vi "IsmaTest_V2.vi"() -> ()   [LabVIEW 2017]
uses:
  BERTTA.dll
panel:
  out "pumpCTRL":dbl
  out "elapsed":dbl
  out "time_to_target":dbl
  out "Boolean 9":bool
  out "Boolean 8":bool
  out "Boolean 7":bool
  out "Boolean 6":bool
  out "Boolean 5":bool
  out "Boolean 4":bool
  out "Boolean 3":bool
  out "Boolean 2":bool
  out "Boolean":bool
  in  "Setpoint_W   /   Setpoint_T":dbl[][](array[numeric])
  in  "Pause":bool
  in  "Reset":bool
  in  "Manual":bool
  in  "Enable":bool
  in  "FR_manual":dbl
  out "FR":dbl(graph)
  out "paramsIn":dbl[](array[numeric])
  out "paramsOut":dbl[](array[numeric])
  out "RPM":dbl
  out "Weight":dbl
  in  "port_isma":i32=7
  in  "port":i32=4
  # "STOP"
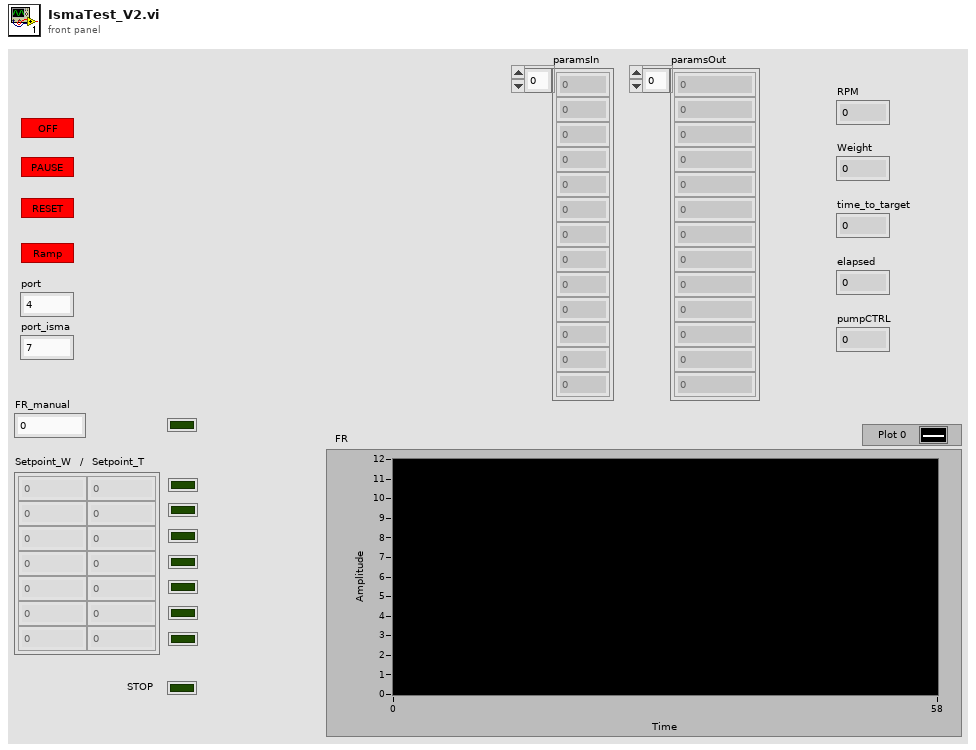
[diagram p1: front panel]
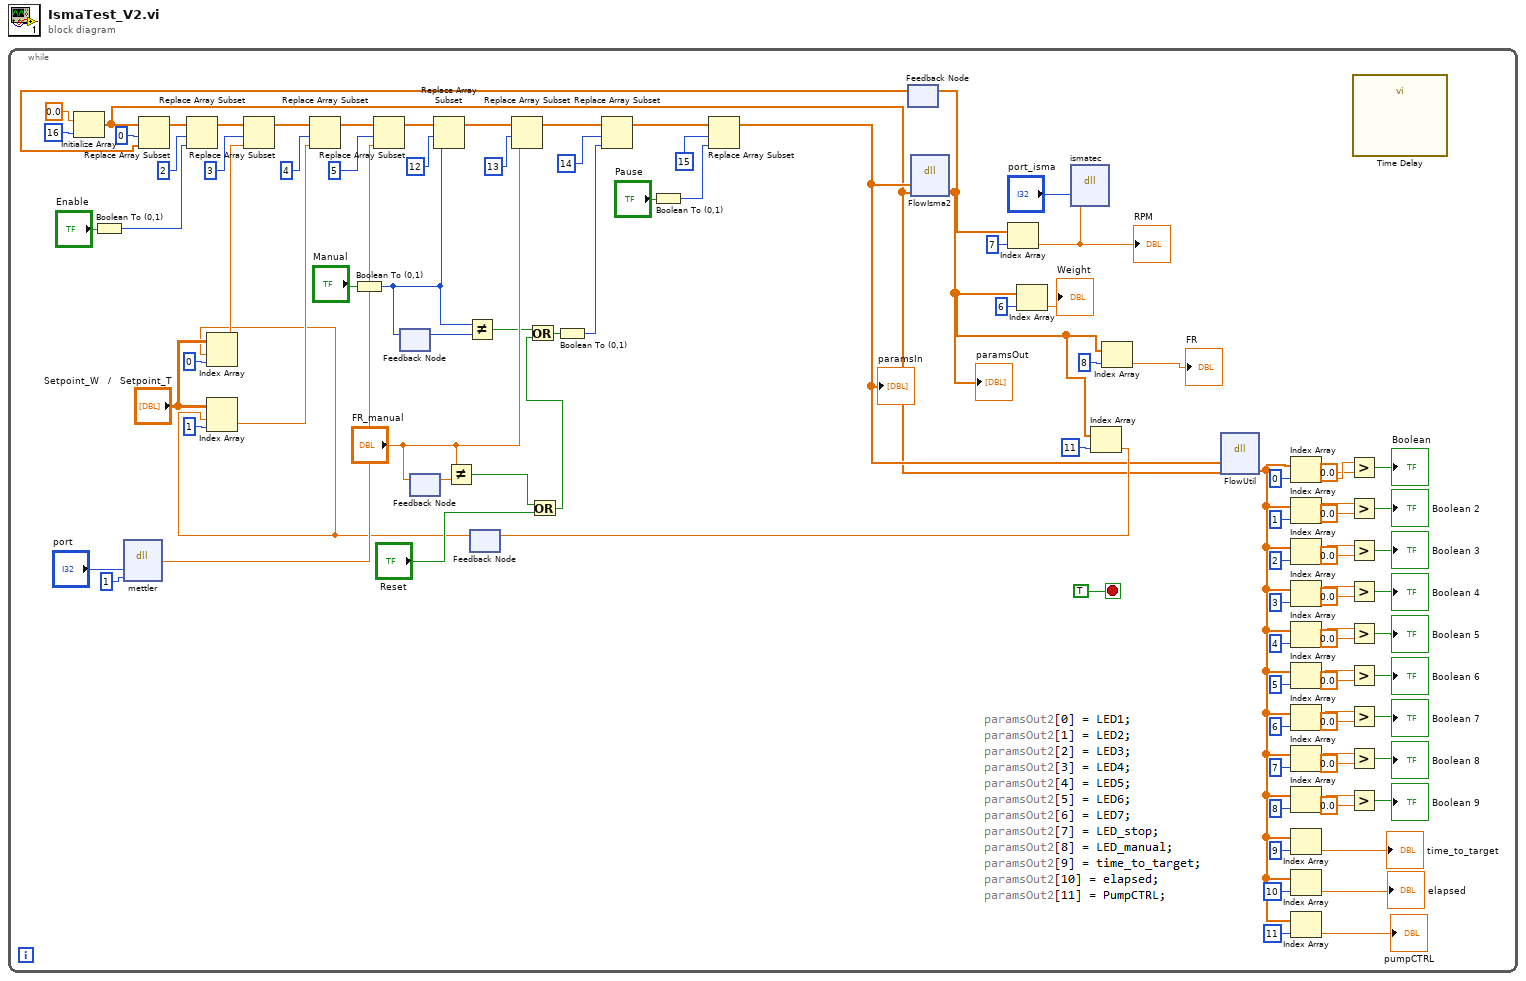
[diagram p0: block diagram]
diagram:
  n1 = while {
    stop <- TRUE stop-if-true
    n2 = Initialize Array(0.0 ("element"), 16 ("dimension size")) -> (w1:dbl[])
    n3 = Boolean To (0,1)(Boolean="Enable") -> (0, 1=w73:i16)
    n4 = dll-call lib="C:/Users/shresplab/OneDrive - Kemira Oyj/Documents/GitHub/Bertta/BERTTA/x64/Debug/BERTTA.dll" fn="mettler"("port"="port", "msg"=1) -> ("return type"=w90:dbl)  [unwired: 5 in, 2 out]
    n5 = Boolean To (0,1)(Boolean="Manual") -> (0, 1=w64:i16)
    n6 = feedback #1() -> (w65:i16)  [unwired: 1 in]
    n7 = feedback-in #1(w64) -> ()
    n8 = feedback #2() -> (w68:dbl)  [unwired: 1 in]
    n9 = feedback-in #2("FR_manual") -> ()
    n10 = Not Equal?(x="FR_manual", y=w68) -> (x != y?=w67:bool)
    n11 = Not Equal?(x=w64, y=w65) -> (x != y?=w61:bool)
    n12 = feedback #3() -> (w46:dbl)  [unwired: 1 in]
    n13 = Index Array(array="Setpoint_W   /   Setpoint_T", index (row)=w46, index (col)=0 ("disabled index (col)")) -> (element=w53:dbl)
    n14 = Index Array(array="Setpoint_W   /   Setpoint_T", index (row)=w46, index (col)=1 ("disabled index (col)")) -> (element=w50:dbl)
    n15 = Or(x=w67, y="Reset") -> (x .or. y?=w60:bool)
    n16 = Or(x=w61, y=w60) -> (x .or. y?=w63:bool)
    n17 = Boolean To (0,1)(Boolean=w63) -> (0, 1=w62:i16)
    n18 = Boolean To (0,1)(Boolean="Pause") -> (0, 1=w55:i16)
    n19 = feedback #4() -> (w82:dbl[])  [unwired: 1 in]
    n20 = Replace Array Subset(array=w1, new element=w82, index=0) -> (w81:dbl[])
    n21 = Replace Array Subset(array=w81, new element=w73, index=2) -> (w95:dbl[])
    n22 = Replace Array Subset(array=w95, new element=w53, index=3) -> (w93:dbl[])
    n23 = Replace Array Subset(array=w93, new element=w50, index=4) -> (w91:dbl[])
    n24 = Replace Array Subset(array=w91, new element=w90, index=5) -> (w78:dbl[])
    n25 = Replace Array Subset(array=w78, new element=w64, index=12) -> (w75:dbl[])
    n26 = Replace Array Subset(array=w75, new element="FR_manual", index=13) -> (w70:dbl[])
    n27 = Replace Array Subset(array=w70, new element=w62, index=14) -> (w57:dbl[])
    n28 = Replace Array Subset(array=w57, new element=w55, index=15) -> (w45:dbl[])
    "paramsIn" <- w45
    n29 = dll-call lib="C:/Users/shresplab/OneDrive - Kemira Oyj/Documents/GitHub/Bertta/BERTTA/x64/Debug/BERTTA.dll" fn="FlowIsma2"("paramsIn"=w45, "paramsOut"=w1) -> ("paramsOut"=w48:dbl[])  [unwired: 5 in, 2 out]
    "paramsOut" <- w48
    n30 = feedback-in #4(w48) -> ()
    n31 = Index Array(array=w48, index=7) -> (element=w86:dbl)
    "RPM" <- w86
    n32 = Index Array(array=w48, index=6) -> (element=→"Weight":dbl)
    n33 = dll-call lib="C:/Users/shresplab/OneDrive - Kemira Oyj/Documents/GitHub/Bertta/BERTTA/x64/Debug/BERTTA.dll" fn="ismatec"("port"="port_isma", "speed"=w86) -> ()  [unwired: 6 in, 2 out]
    n34 = Index Array(array=w48, index=11) -> (element=w47:dbl)
    n35 = feedback-in #3(w47) -> ()
    n36 = Index Array(array=w48, index=8) -> (element=→"FR":dbl)
    n37 = dll-call lib="C:/Users/shresplab/OneDrive - Kemira Oyj/Documents/GitHub/Bertta/BERTTA/x64/Debug/BERTTA.dll" fn="FlowUtil"("paramsIn"=w45, "paramsOut2"=w1) -> ("paramsOut2"=w32:dbl[])  [unwired: 5 in, 2 out]
    n38 = Index Array(array=w32, index=0) -> (element=w31:dbl)
    n39 = Index Array(array=w32, index=1) -> (element=w30:dbl)
    n40 = Index Array(array=w32, index=2) -> (element=w29:dbl)
    n41 = Index Array(array=w32, index=3) -> (element=w28:dbl)
    n42 = Index Array(array=w32, index=4) -> (element=w27:dbl)
    n43 = Index Array(array=w32, index=5) -> (element=w26:dbl)
    n44 = Index Array(array=w32, index=6) -> (element=w25:dbl)
    n45 = Index Array(array=w32, index=7) -> (element=w24:dbl)
    n46 = Index Array(array=w32, index=8) -> (element=w23:dbl)
    n47 = Index Array(array=w32, index=9) -> (element=→"time_to_target":dbl)
    n48 = Index Array(array=w32, index=10) -> (element=→"elapsed":dbl)
    n49 = Index Array(array=w32, index=11) -> (element=→"pumpCTRL":dbl)
    n50 = Greater?(x=w31, y=0.0) -> (0:→"Boolean":bool)
    n51 = Greater?(x=w30, y=0.0) -> (0:→"Boolean 2":bool)
    n52 = Greater?(x=w29, y=0.0) -> (0:→"Boolean 3":bool)
    n53 = Greater?(x=w28, y=0.0) -> (0:→"Boolean 4":bool)
    n54 = Greater?(x=w27, y=0.0) -> (0:→"Boolean 5":bool)
    n55 = Greater?(x=w26, y=0.0) -> (0:→"Boolean 6":bool)
    n56 = Greater?(x=w25, y=0.0) -> (0:→"Boolean 7":bool)
    n57 = Greater?(x=w24, y=0.0) -> (0:→"Boolean 8":bool)
    n58 = Greater?(x=w23, y=0.0) -> (0:→"Boolean 9":bool)
    n59 = call "Time Delay"() -> ()  [unwired: 11 in, 1 out]
  }
